vi "labview RX Code.vi"() -> ()   [LabVIEW 2014]
uses:
  <vilib>/Instr/_visa.llb/VISA Configure Serial Port (Instr).vi
  <userlib>/_OpenG.lib/labpython/labpython.llb/PYTHON Set Integer Data__ogtk.vi
  <userlib>/_OpenG.lib/labpython/labpython.llb/PYTHON Set Float Data__ogtk.vi
  <userlib>/_OpenG.lib/labpython/labpython.llb/PYTHON Get Integer Data__ogtk.vi
panel:
  in  "key":dbl
  out "error out 2":errorcluster
  in  "decrypt Python script":string
  in  "error in (no error) 2":errorcluster
  in  "VISA resource name":refnum<visa-resource-name>
  in  "error in (no error)":errorcluster
  out "error out":errorcluster
  in  "stop":bool
  out "binarycode":string
  in  "timeout (100 ms)":u32=10000
  in  "baud rate (115200)":u32=9600
  in  "data bits (8)":u16=8 min=5 max=8 step=1
  in  "parity (0:none)":enum16{"None", "Odd", "Even", "Mark", "Space"}(ring)
  in  "flow control (0:none)":u16(ring) items=["None", "XON/XOFF", "RTS/CTS", "XON/XOFF & RTS/CTS", "DTR/DSR", "XON/XOFF & DTR/DSR"]
  in  "stop bits (10: 1 bit)":u16(ring)=10 items=["1.0"=10, "1.5"=15, "2.0"=20]
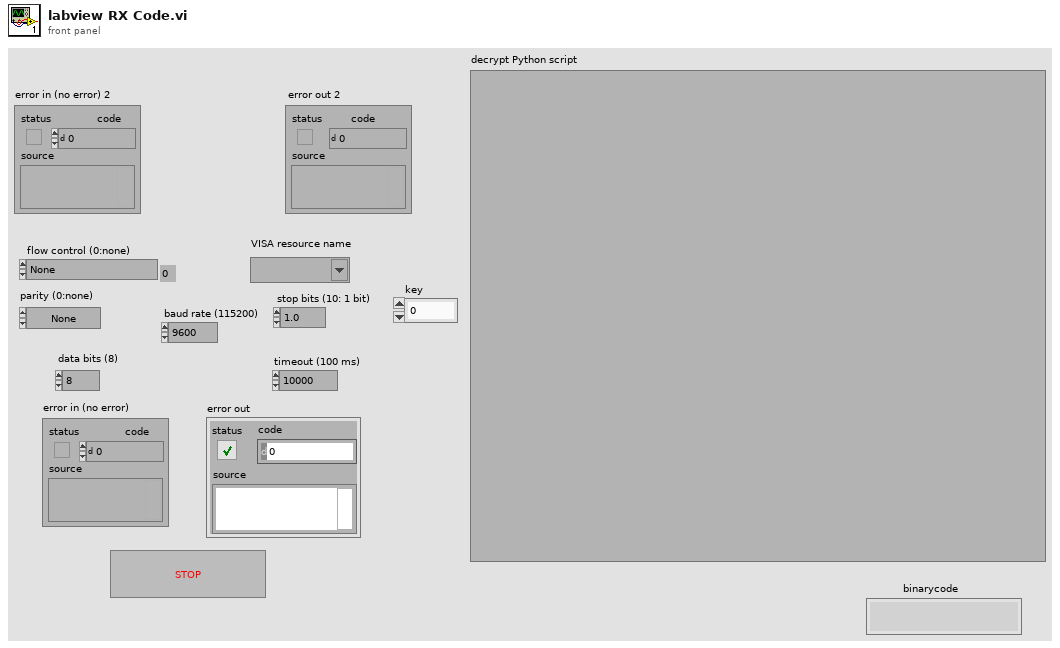
[diagram p1: front panel]
types:
  T1 = typedef "PYTHON Session Refnum__ogtk.ctl" = refnum<k1>
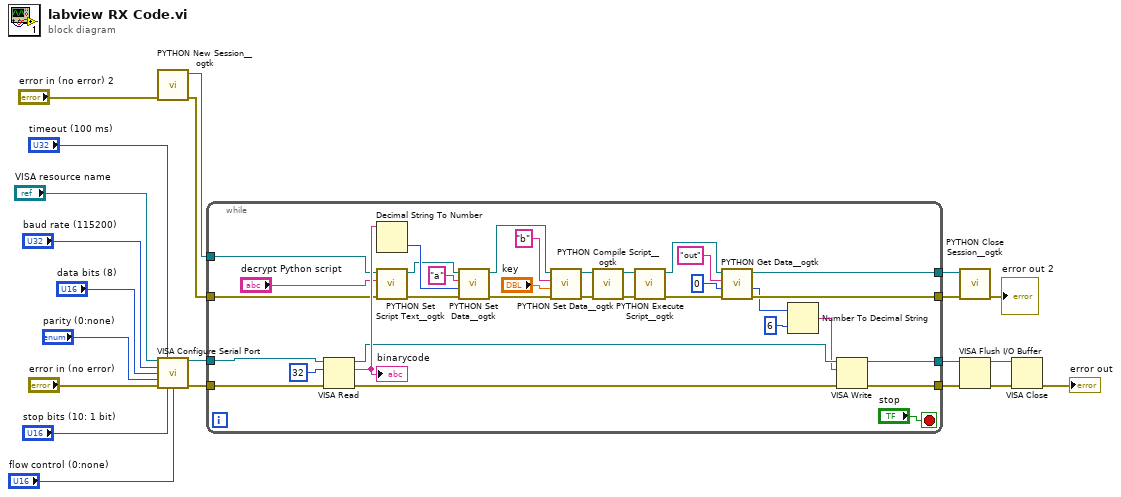
[diagram p0: block diagram]
diagram:
  n1 = call <userlib>:"PYTHON New Session__ogtk.vi"("error in (no error)"="error in (no error) 2") -> ("error out"=w4:errorcluster, "Python Session"=w5:T1)  [unwired: 5 in]
  n2 = call-poly "VISA Configure Serial Port"("VISA resource name"="VISA resource name", "timeout (10sec)"="timeout (100 ms)", "baud rate (9600)"="baud rate (115200)", "data bits (8)"="data bits (8)", "parity (0:none)"="parity (0:none)", "error in (no error)"="error in (no error)", "stop bits (10: 1 bit)"="stop bits (10: 1 bit)", "flow control (0:none)"="flow control (0:none)") -> ("VISA resource name out"=w13:refnum<visa-resource-name>, "error out"=w14:errorcluster)  [unwired: 6 in]
  n3 = while {
    tunnel: w13 -> [w23]
    tunnel: w14 -> [w22]
    tunnel: [w33] -> w20
    tunnel: [w35] -> w18
    tunnel: w5 -> [w43]
    tunnel: w4 -> [w51]
    tunnel: [w45] -> w3
    tunnel: [w44] -> w2
    stop <- "stop" stop-if-true
    n4 = VISA Read(VISA resource name=w23, byte count=32, error in (no error)=w22) -> (VISA resource name out=w36:refnum<visa-resource-name>, read buffer=w52:string, error out=w34:errorcluster)  [unwired: 1 out]
    "binarycode" <- w52
    n5 = Decimal String To Number(string=w52) -> (number=w41:i32)  [unwired: 2 in, 1 out]
    n6 = call <userlib>:"PYTHON Set Script Text__ogtk.vi"("error in (no error)"=w51, "script text"="decrypt Python script", "Python Session in"=w43) -> ("error out"=w50:errorcluster, "Python Session out"=w39:T1)  [unwired: 3 in]
    n7 = call-poly <userlib>:"PYTHON Set Data__ogtk.vi"("error in (no error)"=w50, "value"=w41, "variable name"="a", "Python Session in"=w39) -> ("error out"=w31:errorcluster, "Python Session out"=w32:T1)  [unwired: 2 in]
    n8 = call-poly <userlib>:"PYTHON Set Data__ogtk.vi"("error in (no error)"=w31, "value"="key", "variable name"="b", "Python Session in"=w32) -> ("error out"=w29:errorcluster, "Python Session out"=w30:T1)  [unwired: 2 in]
    n9 = call <userlib>:"PYTHON Compile Script__ogtk.vi"("error in (no error)"=w29, "Python Session in"=w30) -> ("error out"=w37:errorcluster, "Python Session out"=w38:T1)  [unwired: 4 in]
    n10 = call <userlib>:"PYTHON Execute Script__ogtk.vi"("error in (no error)"=w37, "Python Session in"=w38) -> ("error out"=w48:errorcluster, "Python Session out"=w49:T1)  [unwired: 4 in]
    n11 = call-poly <userlib>:"PYTHON Get Data__ogtk.vi"("error in (no error)"=w48, "data type"=0, "variable name"="out", "Python Session in"=w49) -> ("error out"=w44:errorcluster, "value"=w26:i32, "Python Session out"=w45:T1)  [unwired: 1 in]
    n12 = Number To Decimal String(number=w26, width (-)=i16 6) -> (decimal integer string=w25:string)
    n13 = VISA Write(VISA resource name=w36, write buffer=w25, error in (no error)=w34) -> (VISA resource name out=w35:refnum<visa-resource-name>, error out=w33:errorcluster)  [unwired: 1 out]
  }
  n14 = call <userlib>:"PYTHON Close Session__ogtk.vi"("error in (no error)"=w2, "Python Session in"=w3) -> ("error out"=→"error out 2":errorcluster)  [unwired: 5 in]
  n15 = VISA Flush I/O Buffer(VISA resource name=w18, error in (no error)=w20) -> (VISA resource name out=w19:refnum<visa-resource-name>, error out=w21:errorcluster)  [unwired: 1 in]
  n16 = VISA Close(VISA resource name=w19, error in (no error)=w21) -> (error out=→"error out":errorcluster)
